vi "Cascade MEMS Only VCmin.vi"(7 "V Bias":dbl, 8 "Error In":errorcluster, 9 "V3":string[](array[string]), 10 "V2":string[](array[string]), 11 "V1":string[](array[string])) -> (0 "Error Out":errorcluster, 3 "VCmin":string[](array[string]))   [LabVIEW 2017]
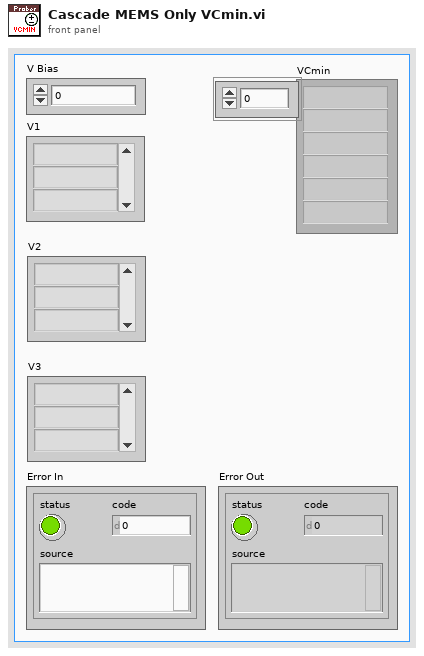
[diagram p1: front panel]
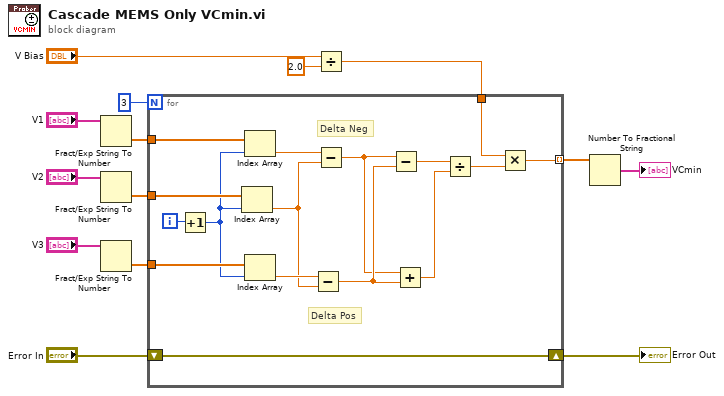
[diagram p0: block diagram]
diagram:
  n1 = Fract/Exp String To Number(string="V1") -> (number=w11:dbl[])  [unwired: 3 in, 1 out]
  n2 = Fract/Exp String To Number(string="V2") -> (number=w9:dbl[])  [unwired: 3 in, 1 out]
  n3 = Fract/Exp String To Number(string="V3") -> (number=w10:dbl[])  [unwired: 3 in, 1 out]
  n4 = Divide(x="V Bias", y=2.0) -> (x/y=w6:dbl)
  n5 = for {
    N: 3 -> [_]
    tunnel: w11 -> [w30]
    tunnel: w10 -> [w29]
    tunnel: w9 -> [w27]
    tunnel: w6 -> [w19]
    tunnel: [w16] -> w4 mode=indexing
    shift-right: [w15] -> w1
    shift-left: "Error In" -> [w15]
    i -> [w18]
    # "Delta Pos"
    # "Delta Neg"
    n6 = Increment(x=w18) -> (x+1=w17:i32)
    n7 = Index Array(array=w27, index=w17) -> (element=w25:dbl)
    n8 = Index Array(array=w30, index=w17) -> (element=w28:dbl)
    n9 = Index Array(array=w29, index=w17) -> (element=w26:dbl)
    n10 = Subtract(x=w26, y=w25) -> (x-y=w24:dbl)
    n11 = Subtract(x=w28, y=w25) -> (x-y=w23:dbl)
    n12 = Subtract(x=w23, y=w24) -> (x-y=w22:dbl)
    n13 = Add(x=w23, y=w24) -> (x+y=w21:dbl)
    n14 = Divide(x=w22, y=w21) -> (x/y=w20:dbl)
    n15 = Multiply(x=w19, y=w20) -> (x*y=w16:dbl)
  }
  "Error Out" <- w1
  n16 = Number To Fractional String(number=w4) -> (F-format string=→"VCmin":string[])  [unwired: 3 in]
